vi "registerAll.vi"(8 "error in (no error)":errorcluster, 11 "SAL_Listener in":refnum<class "SAL_Listener.lvclass">) -> (0 "error out":errorcluster, 3 "SAL_Listener out":refnum<class "SAL_Listener.lvclass">)   [LabVIEW 2016, in "SAL_Listener.lvclass"]
uses:
  SAL_Listener.lvclass
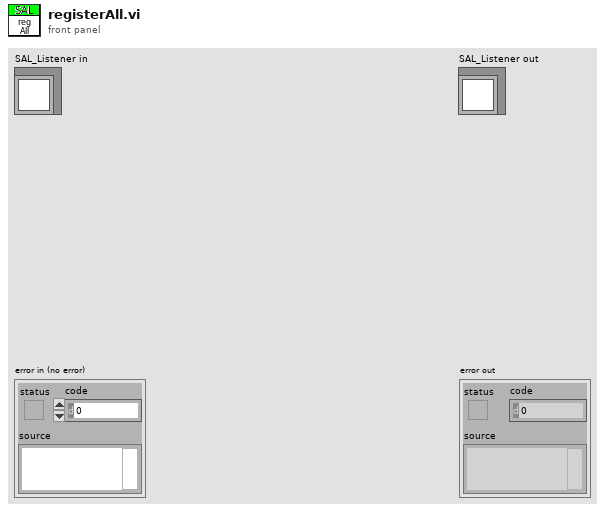
[diagram p1: front panel]
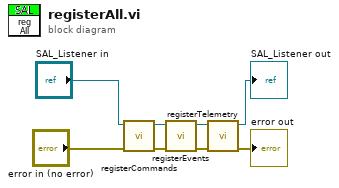
[diagram p0: block diagram]
diagram:
  n1 = call "registerCommands.vi"("error in (no error)"="error in (no error)", "SAL_Listener in"="SAL_Listener in") -> ("error out"=w7:errorcluster, "SAL_Listener out"=w8:refnum<class "SAL_Listener.lvclass">)  [unwired: 8 in]
  n2 = call "registerEvents.vi"("error in (no error)"=w7, "SAL_Listener in"=w8) -> ("error out"=w6:errorcluster, "SAL_Listener out"=w5:refnum<class "SAL_Listener.lvclass">)  [unwired: 8 in]
  n3 = call "registerTelemetry.vi"("error in (no error)"=w6, "SAL_Listener in"=w5) -> ("error out"=→"error out":errorcluster, "SAL_Listener out"=→"SAL_Listener out":refnum<class "SAL_Listener.lvclass">)  [unwired: 8 in]
